vi "iWorx Light & Laser SubVI (Linear).vi"(7 "# of Timestamps to store (10)":u32=10, 9 "Threasholds (1V)":dbl[](array[numeric])=[1.0, 1.0], 11 "Waveform Array":waveform(dbl)[](array[waveform])) -> (1 "Ch 2 Beam Break Duration (s)":dbl, 2 "Ch 1 Beam Break Duration (s)":dbl, 3 "Two Edge Seperation (s)":dbl, 4 "Edge Times":T1, 5 "Raw Signal":cluster{dbl, dbl}(knob)={0.0, 1.7621809600690803} scale=-5.0..5.0)   [LabVIEW 2012]
doc: "This sub VI takes an <b>Array of Waveforms</b> read from the iWorx Light & Laser sensor (x2) set up in a linear photogate. It returns the <b>Beam Break Duration</b> so you calculate speed based the length of an object and the <b>Two Edge Separation</b> so you can calculate speed based on the distance between the two sets of sensors. For positive times set up the beams so Channel 1 is crossed first."
uses:
  <vilib>/ptbypt/NI_PtbyPt.lvlib
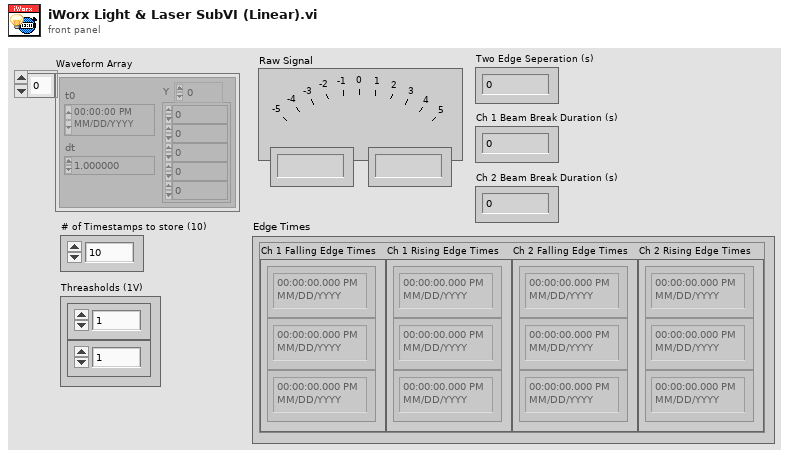
[diagram p1: front panel]
types:
  T1 = cluster{"Ch 1 Falling Edge Times":timestamp[], "Ch 1 Rising Edge Times":timestamp[], "Ch 2 Falling Edge Times":timestamp[], "Ch 2 Rising Edge Times":timestamp[]}
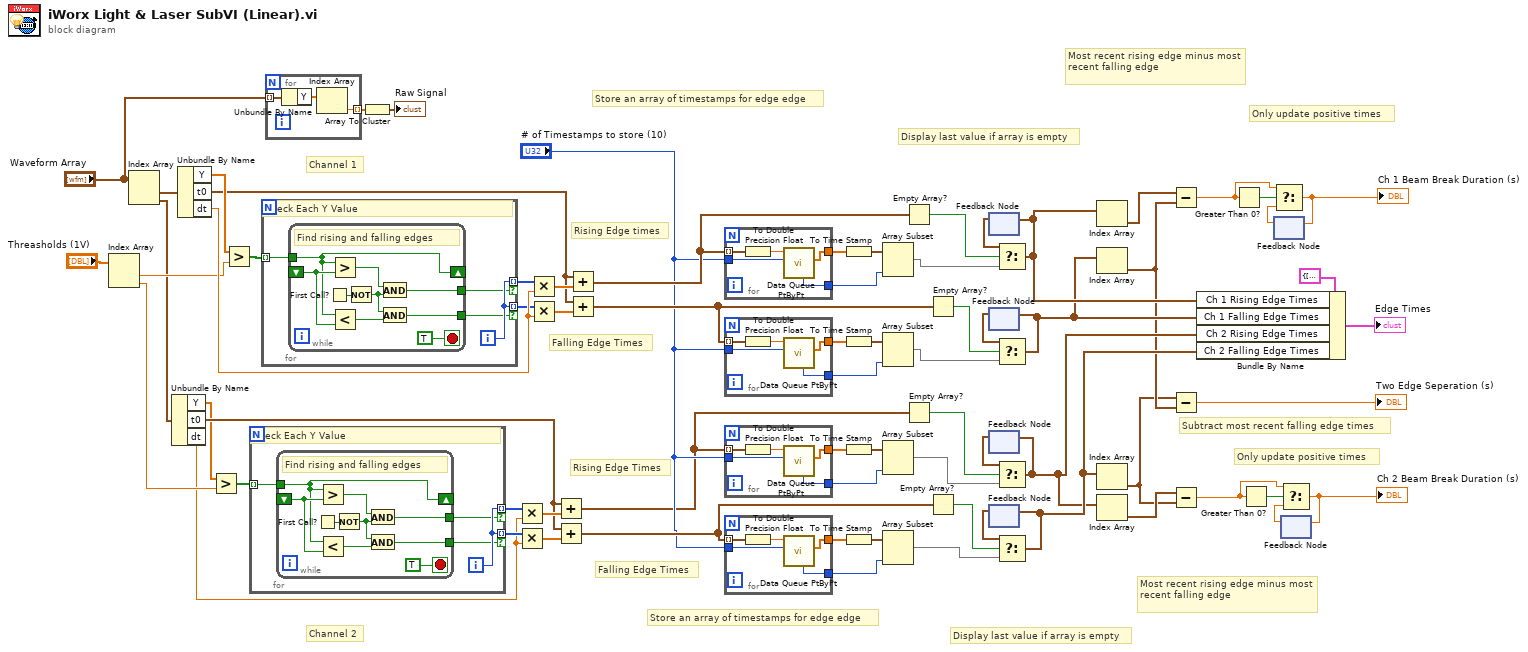
[diagram p0: block diagram]
diagram:
  # "Subtract most recent falling edge times"
  # "Display last value if array is empty"
  # "Store an array of timestamps for edge edge"
  # "Only update positive times"
  # "Only update positive times"
  # "Most recent rising edge minus most recent falling edge"
  # "Most recent rising edge minus most recent falling edge"
  # "Falling Edge Times"
  # "Rising Edge Times"
  # "Channel 2"
  # "Channel 1"
  # "Display last value if array is empty"
  # "Falling Edge Times"
  # "Rising Edge times"
  # "Store an array of timestamps for edge edge"
  n1 = Index Array(array="Threasholds (1V)") -> (element #1=w55:dbl, element #2=w51:dbl)  [unwired: 2 in]
  n2 = Index Array(array="Waveform Array") -> (element #1=w60:waveform(dbl), element #2=w52:waveform(dbl))  [unwired: 2 in]
  n3 = Unbundle By Name(w52) -> ("Y"=w53:dbl[], "t0"=w54:timestamp, "dt"=w49:dbl)
  n4 = Unbundle By Name(w60) -> ("Y"=w65:dbl[], "t0"=w62:timestamp, "dt"=w67:dbl)
  n5 = Greater?(x=w53, y=w51) -> (0:w50:bool[])
  n6 = Greater?(x=w65, y=w55) -> (0:w64:bool[])
  n7 = for {
    tunnel: [w76] -> w57 mode=indexing if=w74
    tunnel: [w76] -> w56 mode=indexing if=w73
    tunnel: w50 -> [w75] mode=indexing
    i -> [w76]
    # "Check Each Y Value"
    n8 = while {
      shift-right: [w79] -> _
      shift-left: _ -> [w84]
      tunnel: w75 -> [w79]
      tunnel: [w78] -> w74
      tunnel: [w77] -> w73
      stop <- TRUE stop-if-true
      # "Find rising and falling edges"
      n9 = First Call?() -> (First Call?: T/F=w80:bool)
      n10 = Greater?(x=w79, y=w84) -> (0:w85:bool)
      n11 = Less?(x=w79, y=w84) -> (x < y?=w83:bool)
      n12 = Not(x=w80) -> (.not. x?=w81:bool)
      n13 = And(x=w85, y=w81) -> (x .and. y?=w77:bool)
      n14 = And(x=w81, y=w83) -> (x .and. y?=w78:bool)
    }
  }
  n15 = for {
    tunnel: [w89] -> w66 mode=indexing if=w87
    tunnel: [w89] -> w68 mode=indexing if=w86
    tunnel: w64 -> [w88] mode=indexing
    i -> [w89]
    # "Check Each Y Value"
    n16 = while {
      shift-right: [w92] -> _
      shift-left: _ -> [w97]
      tunnel: w88 -> [w92]
      tunnel: [w91] -> w87
      tunnel: [w90] -> w86
      stop <- TRUE stop-if-true
      # "Find rising and falling edges"
      n17 = First Call?() -> (First Call?: T/F=w93:bool)
      n18 = Greater?(x=w92, y=w97) -> (0:w98:bool)
      n19 = Less?(x=w92, y=w97) -> (x < y?=w96:bool)
      n20 = Not(x=w93) -> (.not. x?=w94:bool)
      n21 = And(x=w98, y=w94) -> (x .and. y?=w90:bool)
      n22 = And(x=w94, y=w96) -> (x .and. y?=w91:bool)
    }
  }
  n23 = for {
    tunnel: "Waveform Array" -> [w101] mode=indexing
    tunnel: [w99] -> w30 mode=indexing
    n24 = Unbundle By Name(w101) -> ("Y"=w100:dbl[])
    n25 = Index Array(array=w100) -> (element=w99:dbl)  [unwired: 1 in]
  }
  n26 = Array To Cluster(array=w30) -> (cluster=→"Raw Signal":cluster{"[0]":dbl, "[1]":dbl})
  n27 = Multiply(x=w56, y=w49) -> (x*y=w58:dbl[])
  n28 = Multiply(x=w57, y=w49) -> (x*y=w59:dbl[])
  n29 = Multiply(x=w68, y=w67) -> (x*y=w63:dbl[])
  n30 = Multiply(x=w66, y=w67) -> (x*y=w61:dbl[])
  n31 = Add(x=w54, y=w58) -> (x+y=w1:timestamp[])
  n32 = Add(x=w54, y=w59) -> (x+y=w5:timestamp[])
  n33 = Add(x=w62, y=w63) -> (x+y=w21:timestamp[])
  n34 = Add(x=w62, y=w61) -> (x+y=w15:timestamp[])
  n35 = for {
    tunnel: w21 -> [w106] mode=indexing
    tunnel: "# of Timestamps to store (10)" -> [w104]
    tunnel: [w102] -> w25
    tunnel: [w103] -> w23
    n36 = To Double Precision Float(number=w106) -> (double precision float=w105:dbl)
    n37 = call <vilib>:"Data Queue PtByPt.vi"("sample length"=w104, "input data point"=w105) -> ("Current Queue"=w102:dbl[], "current length"=w103:i32)  [unwired: 5 in, 3 out]
  }
  n38 = for {
    tunnel: w15 -> [w111] mode=indexing
    tunnel: "# of Timestamps to store (10)" -> [w109]
    tunnel: [w107] -> w17
    tunnel: [w108] -> w19
    n39 = To Double Precision Float(number=w111) -> (double precision float=w110:dbl)
    n40 = call <vilib>:"Data Queue PtByPt.vi"("sample length"=w109, "input data point"=w110) -> ("Current Queue"=w107:dbl[], "current length"=w108:i32)  [unwired: 5 in, 3 out]
  }
  n41 = for {
    tunnel: w1 -> [w116] mode=indexing
    tunnel: "# of Timestamps to store (10)" -> [w114]
    tunnel: [w112] -> w8
    tunnel: [w113] -> w10
    n42 = To Double Precision Float(number=w116) -> (double precision float=w115:dbl)
    n43 = call <vilib>:"Data Queue PtByPt.vi"("sample length"=w114, "input data point"=w115) -> ("Current Queue"=w112:dbl[], "current length"=w113:i32)  [unwired: 5 in, 3 out]
  }
  n44 = for {
    tunnel: w5 -> [w121] mode=indexing
    tunnel: "# of Timestamps to store (10)" -> [w119]
    tunnel: [w117] -> w13
    tunnel: [w118] -> w11
    n45 = To Double Precision Float(number=w121) -> (double precision float=w120:dbl)
    n46 = call <vilib>:"Data Queue PtByPt.vi"("sample length"=w119, "input data point"=w120) -> ("Current Queue"=w117:dbl[], "current length"=w118:i32)  [unwired: 5 in, 3 out]
  }
  n47 = To Time Stamp(1:w25) -> (0:w24:timestamp[])
  n48 = To Time Stamp(1:w17) -> (0:w18:timestamp[])
  n49 = To Time Stamp(1:w8) -> (0:w9:timestamp[])
  n50 = To Time Stamp(1:w13) -> (0:w12:timestamp[])
  n51 = Array Subset(array=w24, length=w23) -> (w20:timestamp[])  [unwired: 1 in]
  n52 = Array Subset(array=w18, length=w19) -> (w16:timestamp[])  [unwired: 1 in]
  n53 = Array Subset(array=w9, length=w10) -> (w6:timestamp[])  [unwired: 1 in]
  n54 = Array Subset(array=w12, length=w11) -> (w2:timestamp[])  [unwired: 1 in]
  n55 = Empty Array?(array=w21) -> (empty?=w22:bool)
  n56 = Empty Array?(array=w1) -> (empty?=w7:bool)
  n57 = Empty Array?(array=w15) -> (empty?=w14:bool)
  n58 = Empty Array?(array=w5) -> (empty?=w3:bool)
  n59 = feedback #1() -> (w72:timestamp[])  [unwired: 1 in]
  n60 = feedback #2() -> (w70:timestamp[])  [unwired: 1 in]
  n61 = feedback #3() -> (w71:timestamp[])  [unwired: 1 in]
  n62 = feedback #4() -> (w69:timestamp[])  [unwired: 1 in]
  n63 = Select(t=w72, s=w22, f=w20) -> (s? t:f=w48:timestamp[])
  n64 = feedback-in #1(w48) -> ()
  n65 = Select(t=w70, s=w14, f=w16) -> (s? t:f=w47:timestamp[])
  n66 = feedback-in #2(w47) -> ()
  n67 = Select(t=w71, s=w7, f=w6) -> (s? t:f=w43:timestamp[])
  n68 = feedback-in #3(w43) -> ()
  n69 = Select(t=w69, s=w3, f=w2) -> (s? t:f=w44:timestamp[])
  n70 = feedback-in #4(w44) -> ()
  n71 = Index Array(array=w48) -> (element=w46:timestamp)  [unwired: 1 in]
  n72 = Index Array(array=w47) -> (element=w37:timestamp)  [unwired: 1 in]
  n73 = Index Array(array=w44) -> (element=w36:timestamp)  [unwired: 1 in]
  n74 = Index Array(array=w43) -> (element=w45:timestamp)  [unwired: 1 in]
  n75 = Subtract(x=w46, y=w37) -> (x-y=w27:dbl)
  n76 = Subtract(x=w36, y=w37) -> (x-y=→"Two Edge Seperation (s)":dbl)
  n77 = Subtract(x=w45, y=w36) -> (x-y=w38:dbl)
  n78 = Bundle By Name(cluster=T1 {"Ch 1 Falling Edge Times"=[], "Ch 1 Rising Edge Times"=[], "Ch 2 Falling Edge Times"=[], "Ch 2 Rising Edge Times"=[]} ("Edge Times 2"), "Ch 1 Rising Edge Times"=w48, "Ch 1 Falling Edge Times"=w47, "Ch 2 Rising Edge Times"=w43, "Ch 2 Falling Edge Times"=w44) -> (→"Edge Times":T1)
  n79 = Greater Than 0?(x=w27) -> (x > 0?=w42:bool)
  n80 = Greater Than 0?(x=w38) -> (x > 0?=w39:bool)
  n81 = feedback #5() -> (w41:dbl)  [unwired: 1 in]
  n82 = Select(t=w27, s=w42, f=w41) -> (s? t:f=w26:dbl)
  "Ch 1 Beam Break Duration (s)" <- w26
  n83 = feedback-in #5(w26) -> ()
  n84 = feedback #6() -> (w40:dbl)  [unwired: 1 in]
  n85 = Select(t=w38, s=w39, f=w40) -> (s? t:f=w32:dbl)
  "Ch 2 Beam Break Duration (s)" <- w32
  n86 = feedback-in #6(w32) -> ()
